vi "FXP NIPLL_CostaLoop.vi"(8 "reset?":bool, 9 "norminal freq [U16.0]":fxp<+,16,0>, 10 "alpha [U16.0]":fxp<+,16,0>, 11 "x[I24.1]":fxp<+/-,24,1>) -> (0 "f":fxp<+/-,32,0> format="%.32g", 1 "z [I32.1]":fxp<+/-,32,1>, 2 "sin(z)":fxp<+/-,16,2> format="%.15g", 3 "cos(z)":fxp<+/-,16,2> format="%.15g")   [LabVIEW 2012]
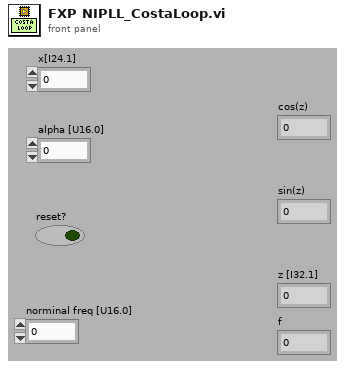
[diagram p1: front panel]
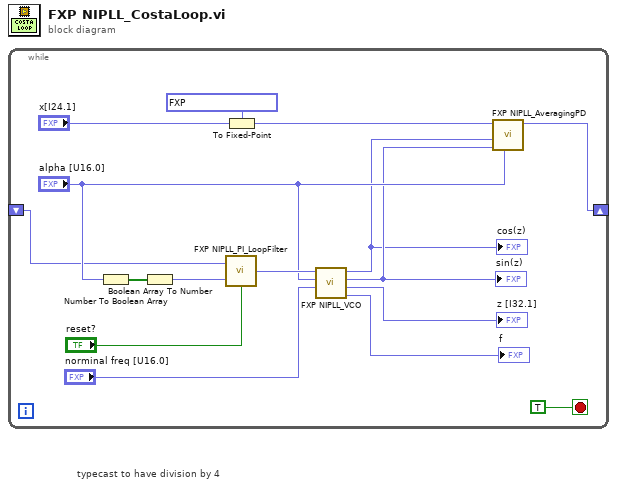
[diagram p0: block diagram]
diagram:
  # "typecast to have division by 4"
  n1 = while {
    shift-right: [w1] -> _
    shift-left: _ -> [w2]
    stop <- TRUE stop-if-true
    n2 = Number To Boolean Array(number="alpha [U16.0]") -> (Boolean array=w12:bool[])
    n3 = Boolean Array To Number(Boolean array=w12) -> (number=w11:fxp<+,16,-2>)
    n4 = call "FXP NIPLL_PI_LoopFilter.vi"("reset?"="reset?", "alpha [U16.-2]"=w11, "x [I16.2]"=w2) -> ("x+y [I48.17]"=w15:fxp<+/-,48,17>)
    n5 = To Fixed-Point(fixed-point type=fxp<+/-,16,1> 0.0 ("number"), number="x[I24.1]") -> (fixed-point=w3:fxp<+/-,16,1>)
    n6 = call "FXP NIPLL_VCO.vi"("nominal freq [U16.0]"="norminal freq [U16.0]", "Kv [U16.0]"="alpha [U16.0]", "v [I48.17]"=w15) -> ("f"=→"f":fxp<+/-,32,0>, "z [I32.1]"=→"z [I32.1]":fxp<+/-,32,1>, "sin(z) [I16.2]"=w7:fxp<+/-,16,2>, "cos(z) [I16.2]"=w6:fxp<+/-,16,2>)  [unwired: 5 in]
    "sin(z)" <- w7
    "cos(z)" <- w6
    n7 = call "FXP NIPLL_AveragingPD.vi"("alpha [U16.0]"="alpha [U16.0]", "sin(z) [I16.2]"=w7, "cos(z) [I16.2]"=w6, "x[I16.1]"=w3) -> ("psd_out"=w1:fxp<+/-,16,2>)  [unwired: 7 in]
  }
